vi "NAttackersPositionPenalty.vi"(0 "N atacantes":u32[](array[numeric]), 1 "Total de n \natacantes":i32, 3 "command\nenum":T1) -> (7 "Posição dos não atacantes\ndurante o penalti":dbl[][](array[numeric]))   [LabVIEW 2017]
uses:
  Command Enum.ctl
panel:
  in  "Array  in":dbl[][](array[numeric])=[[99999.0, 99999.0], [99999.0, 99999.0], [99999.0, 99999.0], [99999.0, 99999.0], [99999.0, 99999.0], [99999.0, 99999.0], [99999.0, 99999.0]]
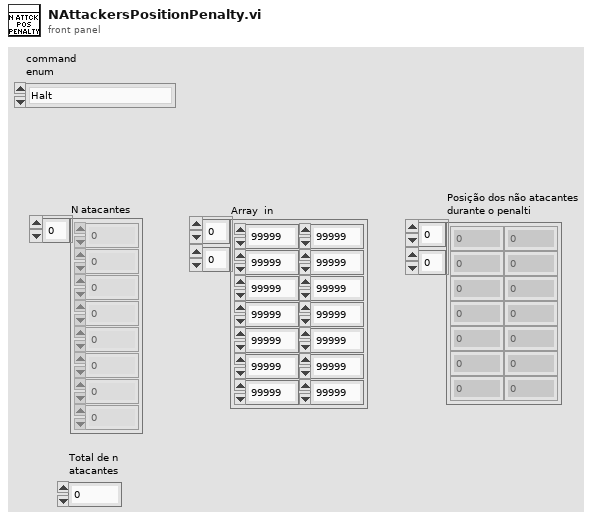
[diagram p1: front panel]
types:
  T1 = typedef "Command Enum.ctl" = enum16{"Halt", "Stop", "Force Start", "PKA Normal Start", "Prepare Kickoff Ally", "PKE Normal Start", "Prepare Kickoff Enemy", "Prepare Penalty Ally", "PPA Normal Start", "Prepare Penalty Enemy", "PPE Normal Start", "Direct Free Enemy", "Direct Free Ally", "Indirect Free Enemy", "Indirect Free Ally", "Timeout Enemy", "Timeout Ally", "Goal Enemy", "Goal Ally", "Ball Placement Enemy", "Ball Placement Ally", "Normal Half Time", "Extra Time Break", "Extra Half Time", "None", "Post Game"}
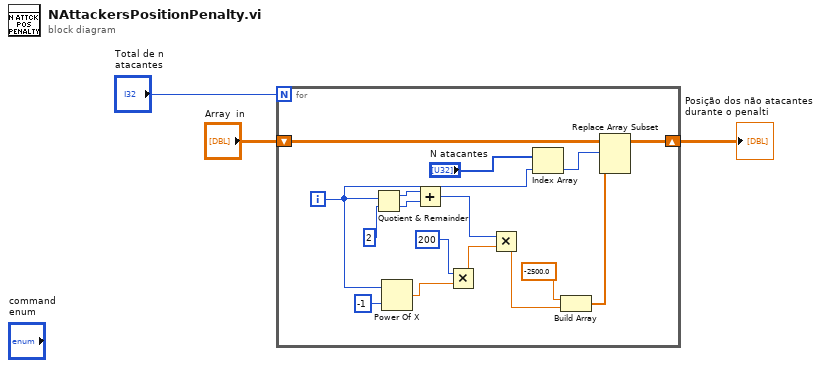
[diagram p0: block diagram]
diagram:
  n1 = for {
    N: "Total de n \natacantes" -> [_]
    shift-right: [w7] -> w3
    shift-left: "Array  in" -> [w8]
    i -> [w5]
    n2 = Quotient & Remainder(x=w5, y=2) -> (x-y*floor(x/y)=w16:i32, floor(x/y)=w15:i32)
    n3 = Power Of X(1:-1 ("x"), 2:w5) -> (0:w18:dbl)
    n4 = Add(x=w16, y=w15) -> (x+y=w14:i32)
    n5 = Multiply(x=200, y=w18) -> (x*y=w13:dbl)
    n6 = Multiply(x=w14, y=w13) -> (x*y=w12:dbl)
    n7 = Index Array(array="N atacantes", index=w5) -> (element=w10:u32)
    n8 = Build Array(-2500.0 ("element"), w12) -> (w6:dbl[])
    n9 = Replace Array Subset(array=w8, new element=w6, index (row)=w10) -> (w7:dbl[][])  [unwired: 1 in]
  }
  "Posição dos não atacantes\ndurante o penalti" <- w3
